vi "Perform LED Test.vi"(8 "error in (no error)":errorcluster, 11 "LCM Single-Up MTS Test in":refnum<class "LCM Single-Up MTS Test.lvclass">) -> (0 "error out":errorcluster, 3 "LED Test Passed":bool)   [LabVIEW 2015, in "LCM Single-Up MTS Test.lvclass"]
uses:
  LCM Single-Up MTS Test.lvclass
  CBTF Applications/SmartCast Testing/Main/LCM Single-Up/Application/Application/Class/typedefs/Instrument Selector -- Enum.ctl
  Classes/Instruments/USB-6001/Class/USB-6001.lvclass
  Classes/Instruments/MIO Device/Class/typedefs/Channel Type -- Enum.ctl
  Classes/Instruments/MIO Device/Class/typedefs/Read Type -- Enum.ctl
  <vilib>/Cree, Inc/Cree Test Framework/Core Launcher/Core Manager Methods -- Enum.ctl
  <vilib>/Analysis/baseanly.llb/Mean (DBL).vi
  <vilib>/Cree, Inc/Cree Test Framework/Classes/Base Objects/Base Class/Base Class/Base Class.lvclass
  Test Class/Test Class.lvclass
  Classes/Application/Class/Application.lvclass
  CBTF Applications/SmartCast Testing/Main/LCM Single-Up/Application/Application/Class/LCM Single-Up.lvclass
  Classes/Manufacturing Test/Class/SC Manufacturing Test.lvclass
  Classes/Test Recipe/Class/Test Recipe.lvclass
  Classes/Instruments/MIO Device/Class/MIO Device.lvclass
  <vilib>/Analysis/NI_AALBase.lvlib
  <vilib>/Cree, Inc/Cree Test Framework/Classes/Data/Data Repo/Class/Data Repo.lvclass
  <vilib>/Cree, Inc/Cree Test Framework/Core Launcher/Core Launcher.lvlib
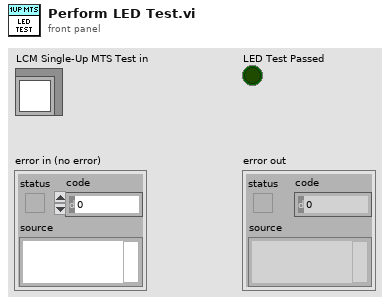
[diagram p1: front panel]
types:
  T1 = typedef "LCM Single-Up.lvlib/LCM Single-Up.lvclass/Instrument Selector -- Enum.ctl" = enum16{"Relay", "MIO Device", "I2C Device", "Thermocouple"}
  T2 = typedef "Application.lvlib/App Properties.lvclass/Class Properties -- Cluster.ctl" = cluster{"UUT Info":T3[], "Test Information":refnum<vi>, "Test Complete Event":refnum<user-event>, "Shop Floor System":refnum<class "Shop Floor System.lvclass">, "Gold Board":refnum<class "Golden Board.lvclass">, "Test Recipe":refnum<class "Test Recipe.lvclass">, "Instruments":refnum<class "Instrument.lvclass">[], "Mode":T4, "Test Results":cluster{"Pass":bool[], "Fail Codes":string[]}, "Station Config":refnum<class "Station Config.lvclass">}
  T3 = typedef "Application.lvlib/App Properties.lvclass/UUT Reference -- Cluster.ctl" = cluster{"Serial Number Reference":refnum<vi>, "Status Message Reference":refnum<vi>}
  T4 = typedef "Application.lvlib/Application.lvclass/Op Mode -- Enum.ctl" = u16
  T5 = typedef "Core Launcher.lvlib/Core Manager Methods -- Enum.ctl" = enum16{"Spawn Objects", "Get Objects", "Destroy Objects"}
  T6 = typedef "MIO Device.lvlib/MIO Device.lvclass/Read Type -- Enum.ctl" = enum16{"Get All", "Get Latest", "Get Average"}
  T7 = typedef "MIO Device.lvlib/MIO Device.lvclass/Channel Type -- Enum.ctl" = enum16{"Analog Input", "Analog Output", "Digital Input", "Digital Output"}
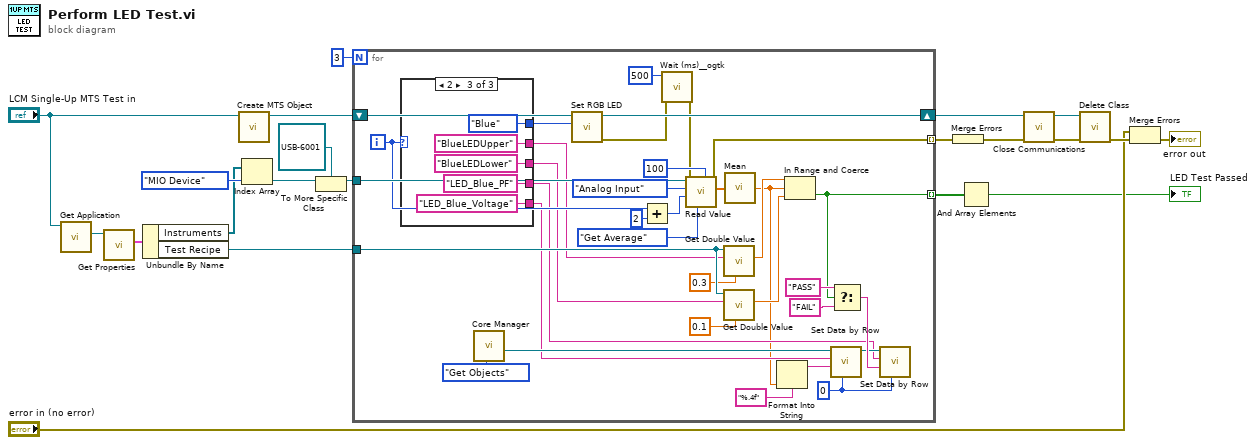
[diagram p0: block diagram]
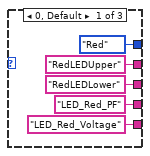
[diagram p2: hidden frame]
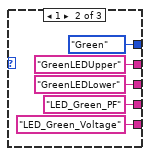
[diagram p3: hidden frame]
diagram:
  n1 = call "Get Application.vi"("Test Class in"="LCM Single-Up MTS Test in") -> ("Application.lvlib:Application.lvclass"=w18:refnum<class "Application.lvclass">)  [unwired: 9 in, 1 out]
  n2 = call "Get Properties.vi"("Acrobat Template in"=w18) -> ("Class Properties"=w17:T2)  [unwired: 8 in, 2 out]
  n3 = Unbundle By Name(w17) -> ("Instruments"=w14:refnum<class "Instrument.lvclass">[], "Test Recipe"=w21:refnum<class "Test Recipe.lvclass">)
  n4 = call "Create MTS Object.vi"("LCM Single-Up MTS Test in"="LCM Single-Up MTS Test in") -> ("MTS"=w13:refnum<class "SC Manufacturing Test.lvclass">)  [unwired: 9 in, 1 out]
  n5 = Index Array(array=w14, index=Instrument_Selector_--_Enum."MIO Device" ("Instrument")) -> (element=w12:refnum<class "Instrument.lvclass">)
  n6 = To More Specific Class(target class=refnum<class "USB-6001.lvclass"> refnum ("Acrobat Template in"), reference=w12) -> (specific class reference=w11:refnum<class "USB-6001.lvclass">)  [unwired: 1 in, 1 out]
  n7 = for {
    N: 3 -> [_]
    tunnel: w21 -> [w55]
    tunnel: w11 -> [w45]
    shift-right: [w46] -> w5
    shift-left: w13 -> [w53]
    tunnel: [w24] -> w9 mode=indexing
    tunnel: [w35] -> w8 mode=indexing
    i -> [w43]
    w32 = 0 ("Row")
    n8 = case shown="2" w43 {
      tunnel: [enum16{"Red", "Green", "Blue"}."Red" ("Color") enum16{"Red", "Green", "Blue"}."Green" ("Color") enum16{"Red", "Green", "Blue"}."Blue" ("Color")] -> w44
      tunnel: ["LED_Red_Voltage" ("Header") "LED_Green_Voltage" ("Header") "LED_Blue_Voltage" ("Header")] -> w33
      tunnel: ["LED_Red_PF" ("Header") "LED_Green_PF" ("Header") "LED_Blue_PF" ("Header")] -> w31
      tunnel: ["RedLEDLower" ("Name") "GreenLEDLower" ("Name") "BlueLEDLower" ("Name")] -> w30
      tunnel: ["RedLEDUpper" ("Name") "GreenLEDUpper" ("Name") "BlueLEDUpper" ("Name")] -> w29
      frame 0, Default {
      }
      frame 1 {
      }
      frame 2 {
      }
    }
    n9 = call <vilib>:"Core Manager.vi"("Method"=Core_Manager_Methods_--_Enum."Get Objects") -> ("Data Repo"=w34:refnum<class "Data Repo.lvclass">)  [unwired: 7 in, 3 out]
    n10 = call "Set RGB LED.vi"("Color"=w44, "Acrobat Template in"=w53) -> ("error out"=w23:errorcluster, "Acrobat Template out"=w46:refnum<class "SC Manufacturing Test.lvclass">)  [unwired: 8 in]
    n11 = Add(x=w43, y=2) -> (x+y=w47:i32)
    n12 = call <userlib>:"Wait (ms)__ogtk.vi"("error in (no error)"=w23, "milliseconds to wait"=u32 500) -> ("error out"=w22:errorcluster)  [unwired: 8 in, 1 out]
    n13 = call-dynamic "Read Value.vi"("Samples to Read (50)"=100, "Read Function (Get All)"=Read_Type_--_Enum."Get Average", "error in (no error)"=w22, "Channel (0)"=w47, "Channel Type"=Channel_Type_--_Enum."Analog Input", "Acrobat Template in"=w45) -> ("error out"=w24:errorcluster, "Value"=w42:dbl[])  [unwired: 3 in, 1 out]
    n14 = call "Get Double Value.vi"("Default Value"=0.3, "Name"=w29, "Test Recipe in"=w55) -> ("Value"=w41:dbl)  [unwired: 6 in, 2 out]
    n15 = call "Get Double Value.vi"("Default Value"=0.1, "Name"=w30, "Test Recipe in"=w55) -> ("Value"=w40:dbl)  [unwired: 6 in, 2 out]
    n16 = call-poly <vilib>:"Mean.vi"("X"=w42) -> ("mean"=w28:dbl)  [unwired: 1 out]
    n17 = Format Into String(format string="%.4f", w28) -> (resulting string=w26:string)  [unwired: 2 in, 1 out]
    n18 = In Range and Coerce(upper limit=w41, x=w28, lower limit=w40) -> (In Range?=w35:bool)  [unwired: 1 out]
    n19 = call <vilib>:"Set Data by Row.vi"("Row"=w32, "Value"=w26, "Header"=w33, "Acrobat Template in"=w34) -> ()  [unwired: 6 in, 2 out]
    n20 = Select(t="PASS" ("Header"), s=w35, f="FAIL" ("Header")) -> (s? t:f=w38:string)
    n21 = call <vilib>:"Set Data by Row.vi"("Row"=w32, "Value"=w38, "Header"=w31, "Acrobat Template in"=w34) -> ()  [unwired: 6 in, 2 out]
  }
  n22 = Merge Errors(w9) -> (w3:errorcluster)
  n23 = And Array Elements(Boolean array=w8) -> (logical AND=→"LED Test Passed":bool)
  n24 = call "Close Communications.vi"("error in (no error)"=w3, "Acrobat Template in"=w5) -> ("error out"=w2:errorcluster, "Acrobat Template out"=w4:refnum<class "SC Manufacturing Test.lvclass">)  [unwired: 8 in]
  n25 = call <vilib>:"Delete Class.vi"("error in (no error)"=w2, "Base Class in"=w4) -> ("error out"=w20:errorcluster)  [unwired: 8 in, 1 out]
  n26 = Merge Errors("error in (no error)", w20) -> (→"error out":errorcluster)
